vi "Initialize Channels.vi"(8 "error in (no error)":errorcluster, 11 "Sift TDMS Uploader in":refnum<class "Sift TDMS Uploader.lvclass">) -> (0 "error out":errorcluster, 3 "Sift TDMS Uploader out":refnum<class "Sift TDMS Uploader.lvclass">)   [LabVIEW 2024, in "Sift TDMS Uploader.lvlib" / "Sift TDMS Uploader.lvclass"]
uses:
  Sift TDMS Uploader.lvclass
  <vilib>/FlexLogger/SDK/PluginSDK.lvlibp/PEFClasses/SDK/Producer Channel/Producer Channel.lvclass
  <vilib>/FlexLogger/SDK/PluginSDK.lvlibp/PEFClasses/SDK/Producer Channel/Create Producer Channel.vi
  Sift TDMS Uploader.lvclass/Sift TDMS Uploader.ctl
  <vilib>/FlexLogger/SDK/PluginSDK.lvlibp/PEFClasses/SDK/Plugin/Plugin.lvclass
  <vilib>/FlexLogger/SDK/PluginSDK.lvlibp
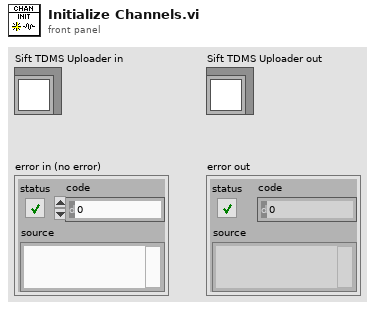
[diagram p1: front panel]
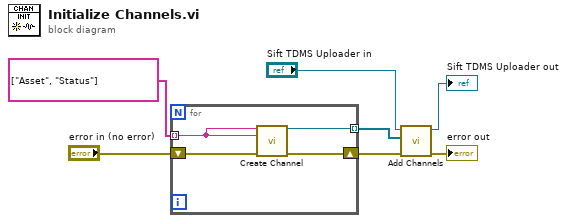
[diagram p0: block diagram]
diagram:
  n1 = for {
    tunnel: [w11] -> w1 mode=indexing
    tunnel: string[] ["Asset", "Status"] -> [w10] mode=indexing
    shift-right: [w8] -> w5
    shift-left: "error in (no error)" -> [w9]
    n2 = call-poly <vilib>:"Create Channel.vi"("Unique Channel Identifier"=w10, "Default Channel Name"=w10, "error in (no error)"=w9) -> ("Producer Channel"=w11:refnum<class "Producer Channel.lvclass">, "error out"=w8:errorcluster)  [unwired: 11 in]
  }
  n3 = call <vilib>:"Add Channels.vi"("error in (no error)"=w5, "Channels"=w1, "Plugin in"="Sift TDMS Uploader in") -> ("error out"=→"error out":errorcluster, "Plugin out"=→"Sift TDMS Uploader out":refnum<class "Sift TDMS Uploader.lvclass">)  [unwired: 7 in]
